vi "MergePaths.vi"(11 "PathArray":T3(array[cluster])) -> (3 "PathOut":T2)   [LabVIEW 2014]
uses:
  TypeDefs/Point2DwSlope.ctl
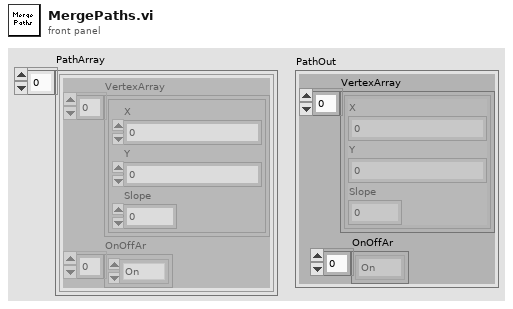
[diagram p1: front panel]
types:
  T1 = typedef "Point2DwSlope.ctl" = cluster{"X":sgl, "Y":sgl, "Slope":dbl}
  T2 = cluster{"VertexArray":T1[], "OnOffAr":enum16{"On", "Off"}[]}
  T3 = cluster{"VertexArray":T1[], "OnOffAr":enum16{"On", "Off"}[]}[]
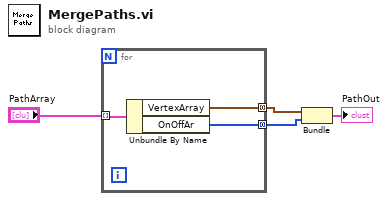
[diagram p0: block diagram]
diagram:
  n1 = for {
    tunnel: "PathArray" -> [w7] mode=indexing
    tunnel: [w6] -> w3 mode=concatenating
    tunnel: [w5] -> w2 mode=concatenating
    n2 = Unbundle By Name(w7) -> ("VertexArray"=w6:T1[], "OnOffAr"=w5:enum16{"On", "Off"}[])
  }
  n3 = Bundle("VertexArray"=w3, "OnOffAr"=w2) -> (→"PathOut":T2)  [unwired: 1 in]
